vi "Subvi trigger delay.vi"(8 "Timeout_tick":u32, 10 "Input":bool) -> (2 "Output":bool)   [LabVIEW 2017]
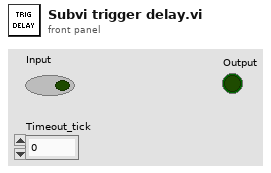
[diagram p1: front panel]
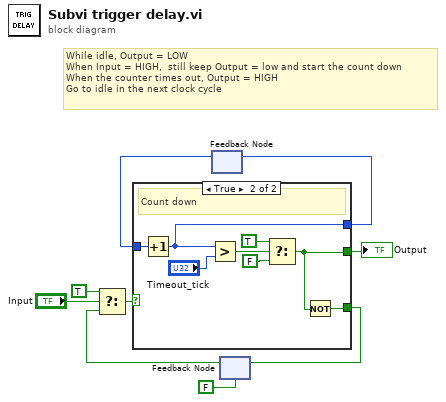
[diagram p0: block diagram]
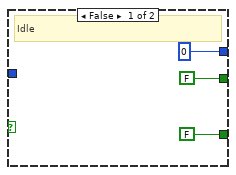
[diagram p2: hidden frame]
diagram:
  # "While idle, Output = LOW\nWhen Input = HIGH,  still keep Output = low and start the count down\nWhen the counter times out, Output = HIGH\nGo to idle in the next clock cycle"
  n1 = feedback #1() -> (w1:u32)  [unwired: 1 in]
  n2 = feedback #2(FALSE) -> (w7:bool)
  n3 = Select(t=TRUE, s="Input", f=w7) -> (s? t:f=w5:bool)
  n4 = case shown="True" w5 {
    tunnel: [FALSE w16] -> w9
    tunnel: [FALSE w17] -> w8
    tunnel: [u32 0 w14] -> w2
    tunnel: w1 -> [_ w15]
    frame False {
      # "Idle"
    }
    frame True {
      # "Count down"
      n5 = Increment(x=w15) -> (x+1=w14:u32)
      n6 = Greater?(x=w14, y="Timeout_tick") -> (0:w18:bool)
      n7 = Select(t=TRUE, s=w18, f=FALSE) -> (s? t:f=w16:bool)
      n8 = Not(x=w16) -> (.not. x?=w17:bool)
    }
  }
  "Output" <- w9
  n9 = feedback-in #1(w2) -> ()
  n10 = feedback-in #2(w8) -> ()
